vi "Read Unique Test ID.vi"(11 "Assert":refnum<class "Assert.lvclass">) -> (2 "Unique Test ID":string, 3 "Assert out":refnum<class "Assert.lvclass">)   [LabVIEW 2013, in "Caraya.lvlib" / "Assert.lvclass"]
uses:
  Assert.lvclass
  Assert.lvclass/Assert.ctl
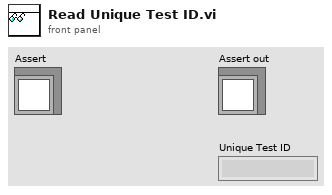
[diagram p1: front panel]
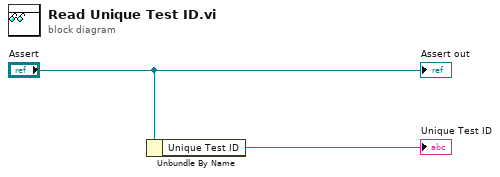
[diagram p0: block diagram]
diagram:
  n1 = Unbundle By Name("Assert") -> ("Unique Test ID"=→"Unique Test ID":string)
  "Assert out" <- "Assert"
